vi "Test Line Result.vi"(5 "Etalon number":u32, 7 "Ignore Error":bool, 8 "error in (no error)":errorcluster, 9 "Teszt cluster":T1, 10 "Thread ID":u16, 11 "Queue in":refnum<queue>) -> (0 "error out":errorcluster, 1 "Abort":bool, 2 "Etalon Kiértékelés":bool, 3 "Kiértékelés":bool)   [LabVIEW 2014]
uses:
  Teszt/Teszt.ctl
  Teszt/Command.ctl
  support/Message Queue/Message Cluster.ctl
  Message.ctl
  support/Message Queue/Enqueue Message (Single).vi
  support/Message Queue/Message Queue.lvlib
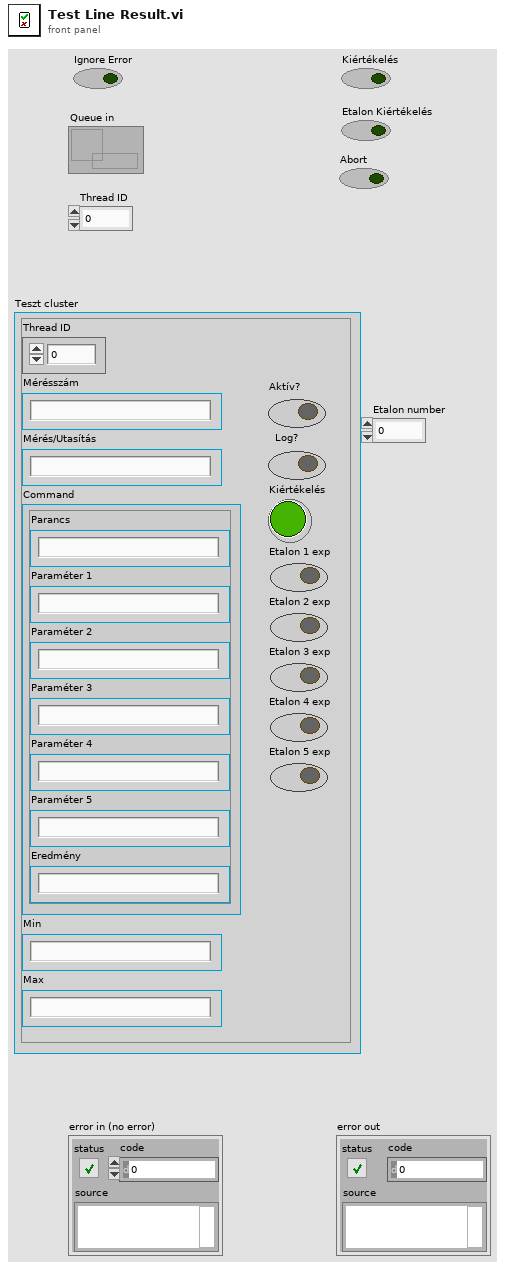
[diagram p1: front panel]
types:
  T1 = typedef "Teszt.ctl" = cluster{"Thread ID":dbl, "Mérésszám":string, "Mérés/Utasítás":string, "Command":T2, "Min":string, "Max":string, "Aktív?":bool, "Log?":bool, "Kiértékelés":bool, "Etalon 1 exp":bool, "Etalon 2 exp":bool, "Etalon 3 exp":bool, "Etalon 4 exp":bool, "Etalon 5 exp":bool}
  T2 = typedef "Command.ctl" = cluster{"Parancs":string, "Paraméter 1":string, "Paraméter 2":string, "Paraméter 3":string, "Paraméter 4":string, "Paraméter 5":string, "Eredmény":string}
  T3 = typedef "Message.ctl" = cluster{"Thread ID":u16, "Callback":string, "Data":variant, "Error":errorcluster}
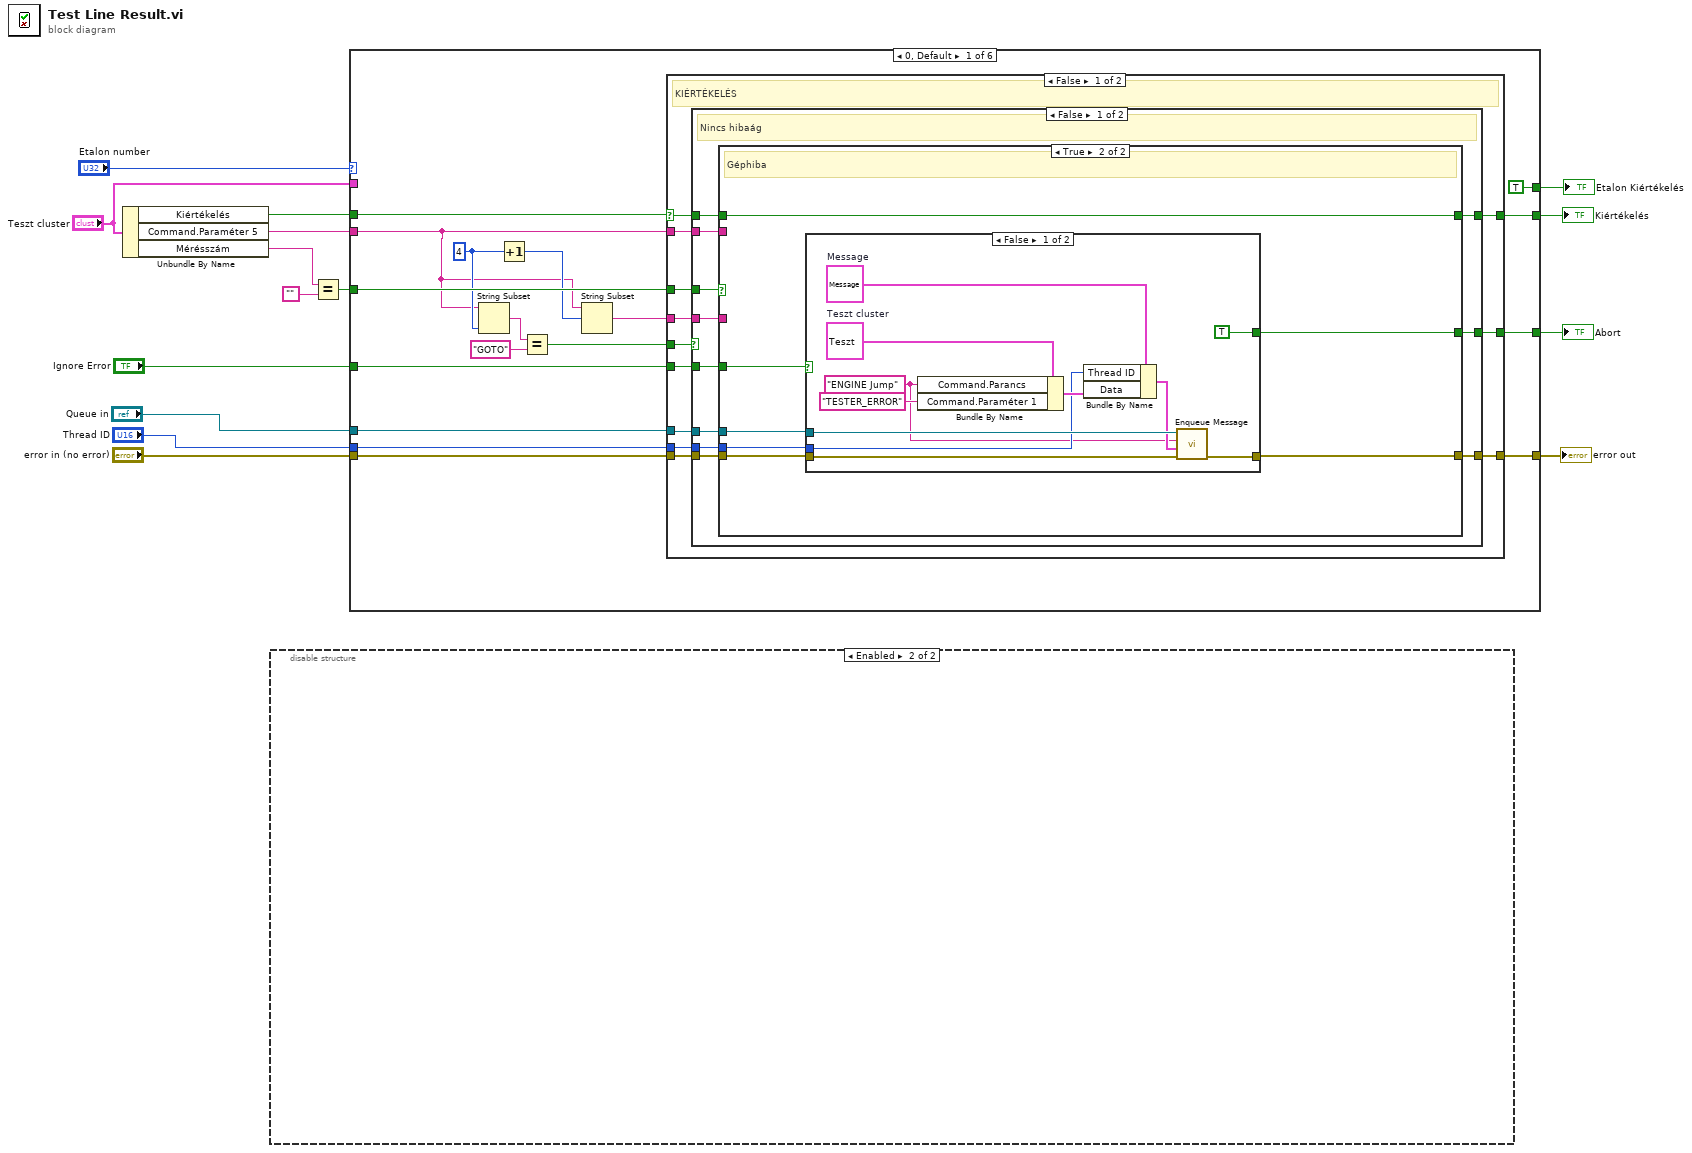
[diagram p0: block diagram]
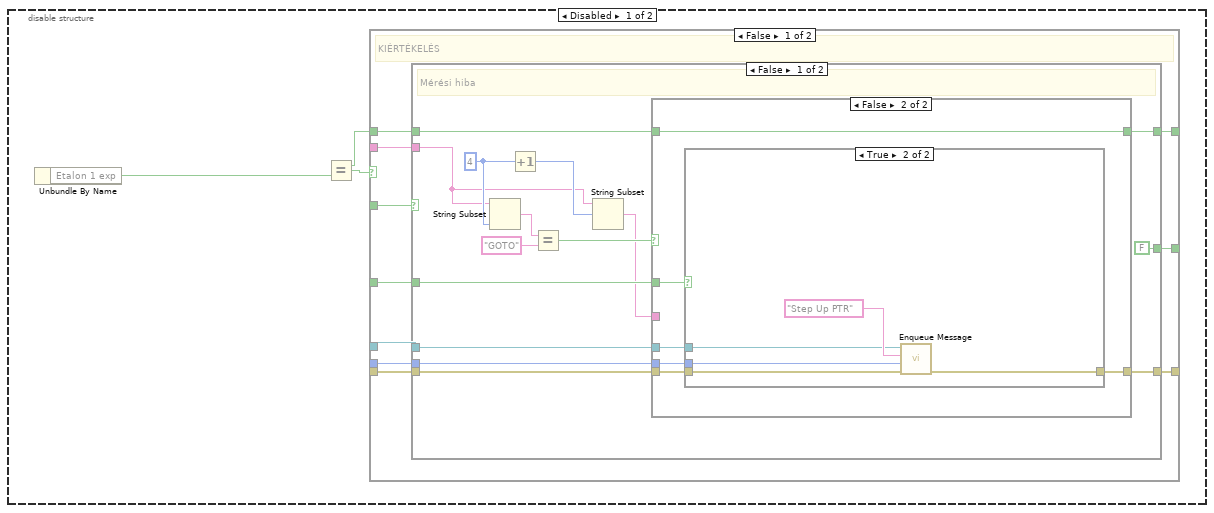
[diagram p2: hidden frame]
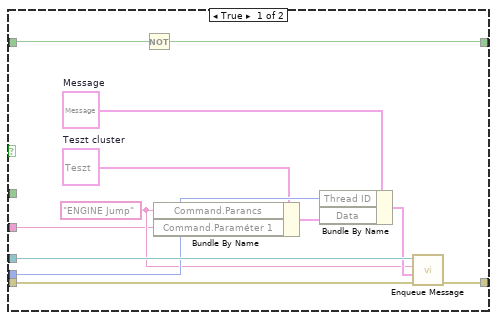
[diagram p3: hidden frame]
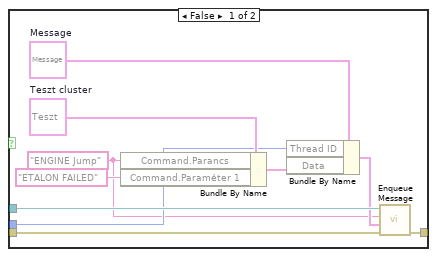
[diagram p4: hidden frame]
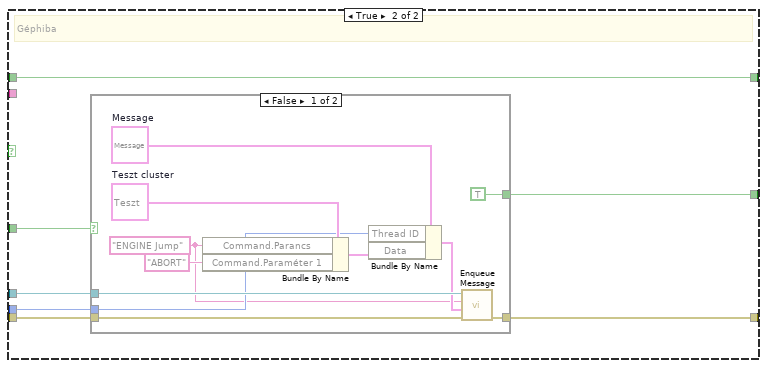
[diagram p5: hidden frame]
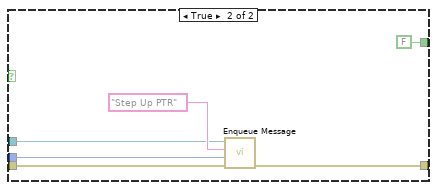
[diagram p6: hidden frame]
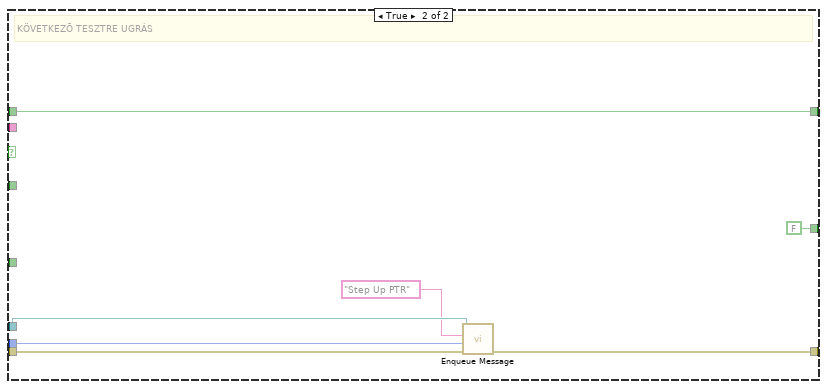
[diagram p7: hidden frame]
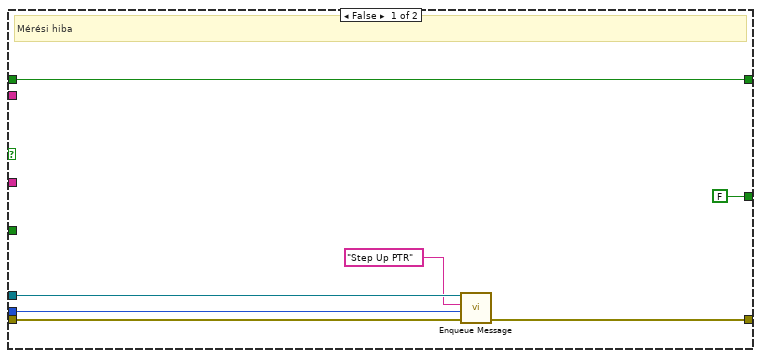
[diagram p8: hidden frame]
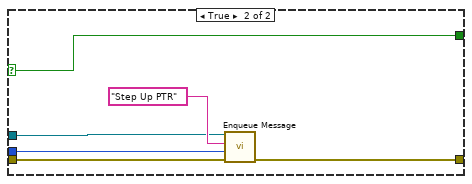
[diagram p9: hidden frame]
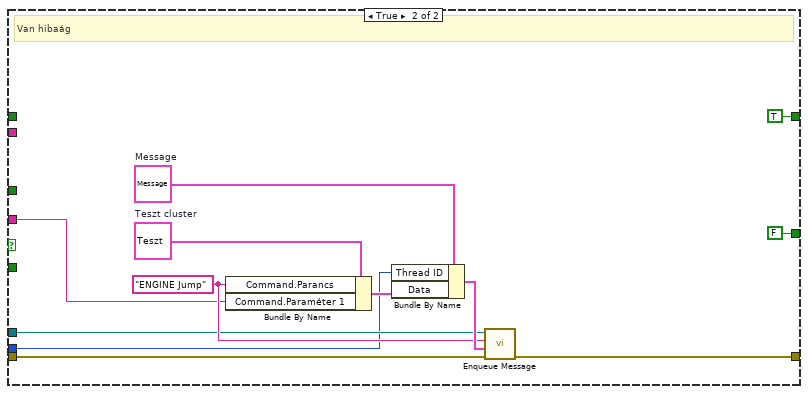
[diagram p10: hidden frame]
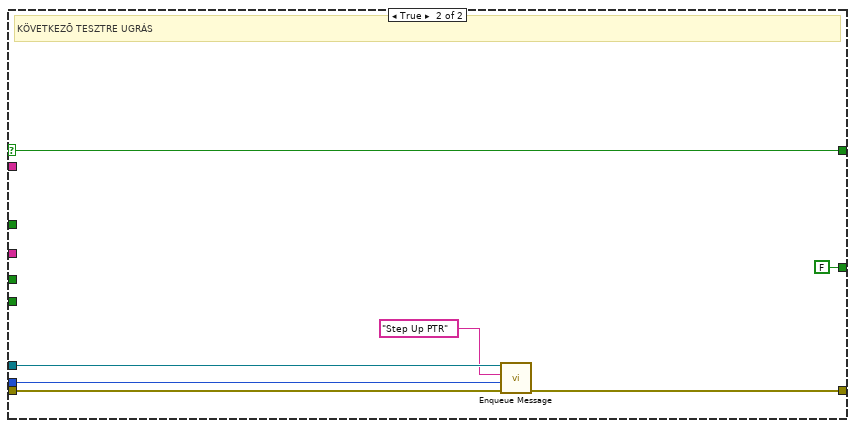
[diagram p11: hidden frame]
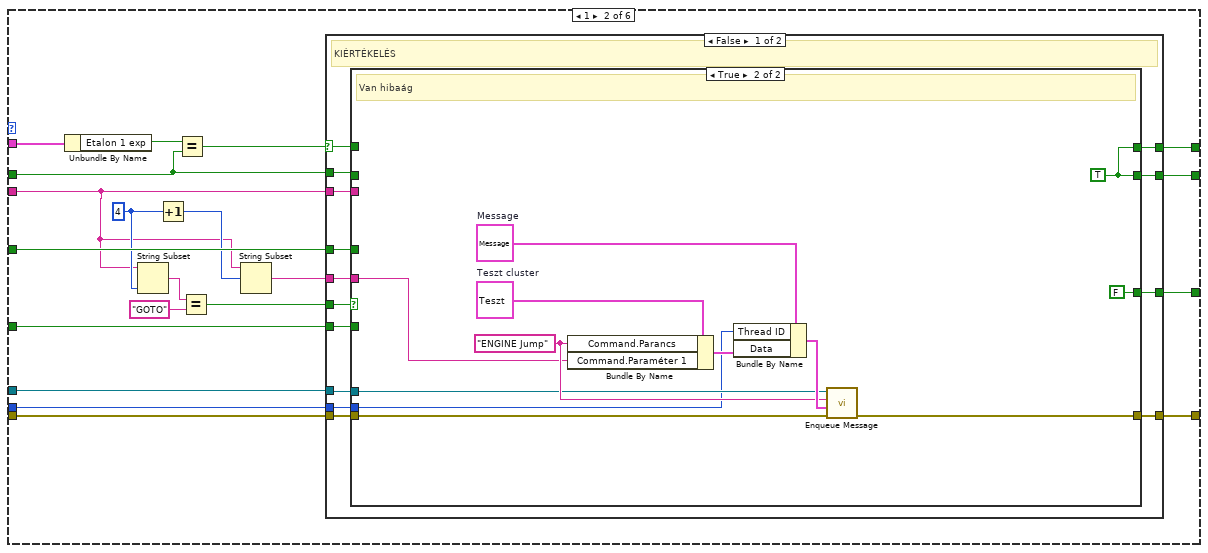
[diagram p12: hidden frame]
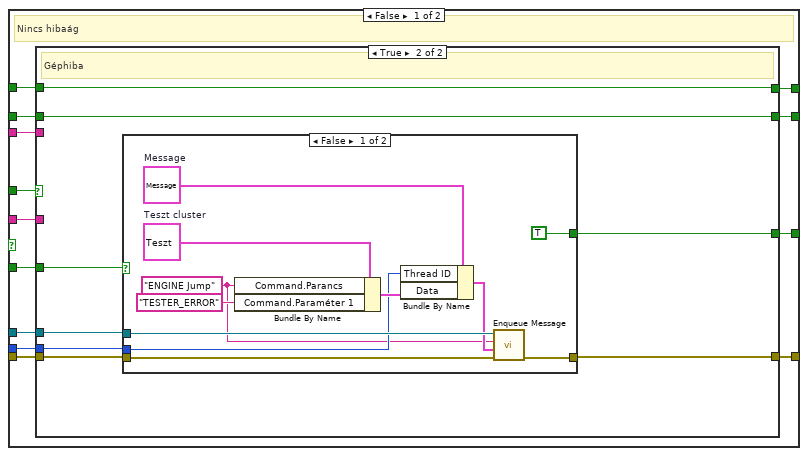
[diagram p13: hidden frame]
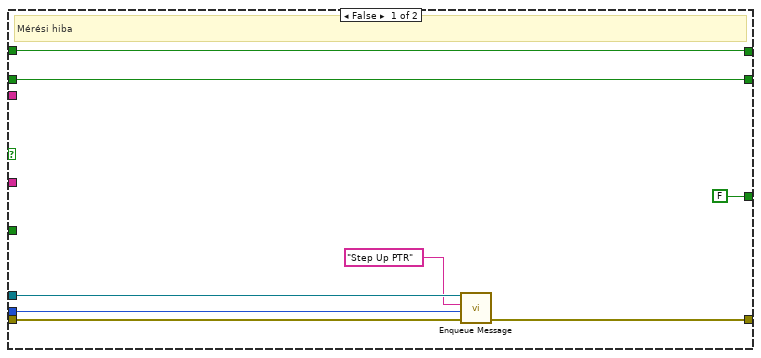
[diagram p14: hidden frame]
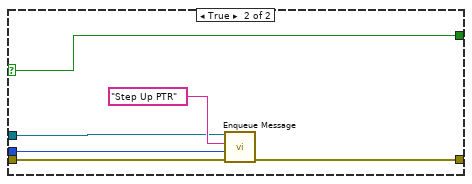
[diagram p15: hidden frame]
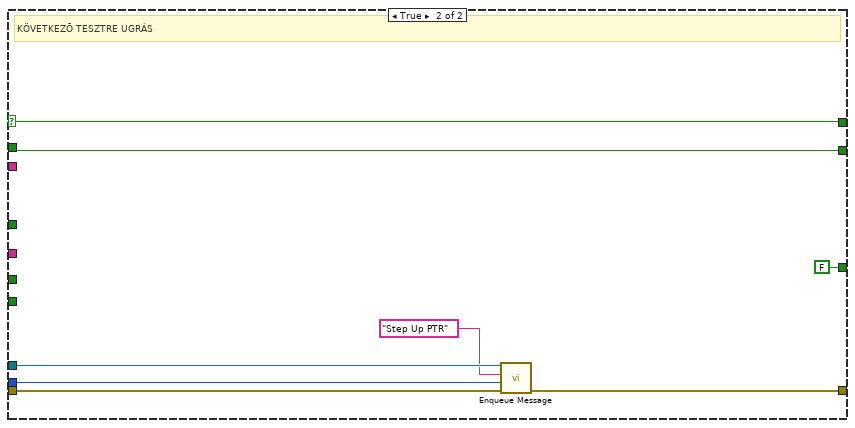
[diagram p16: hidden frame]
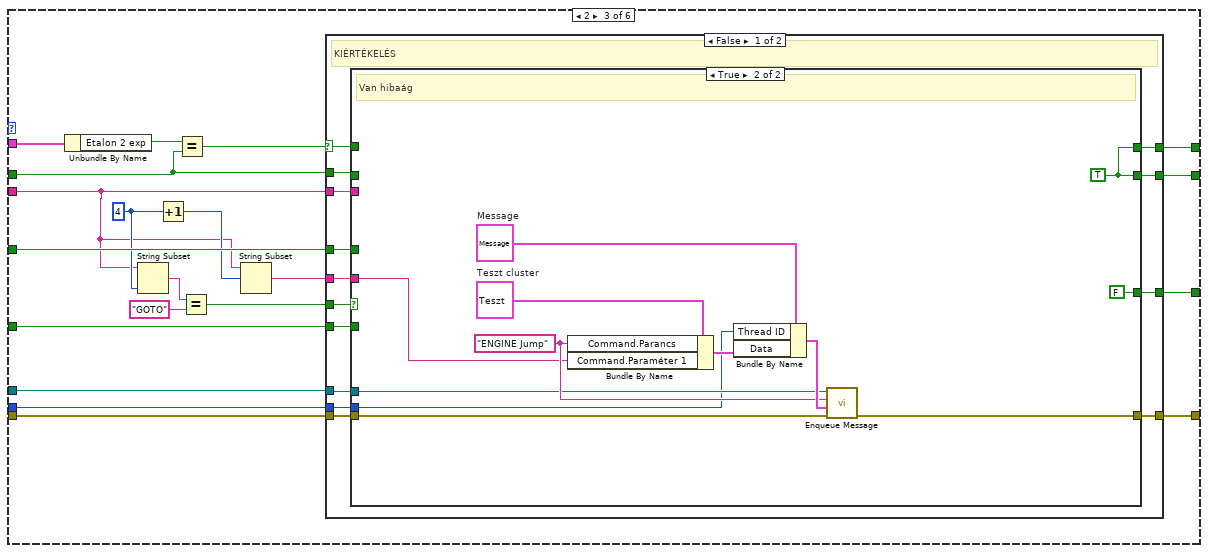
[diagram p17: hidden frame]
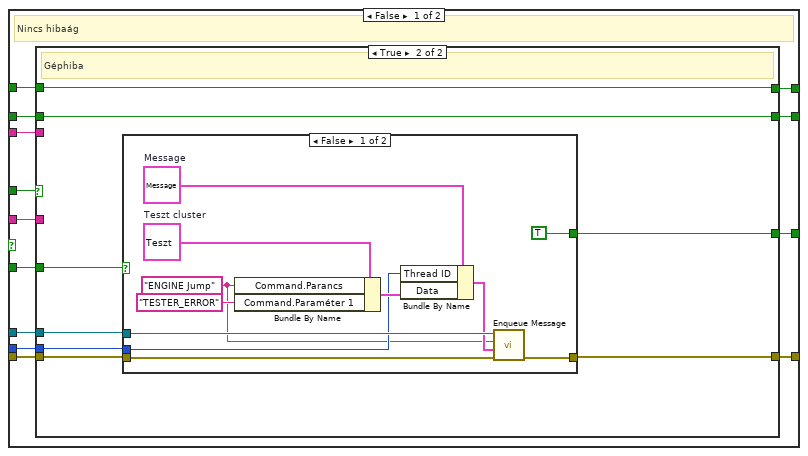
[diagram p18: hidden frame]
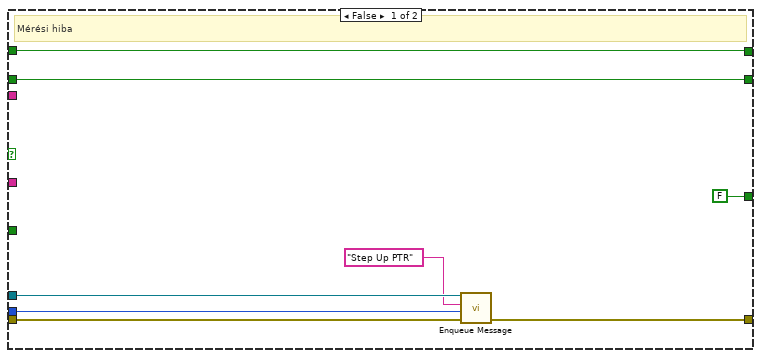
[diagram p19: hidden frame]
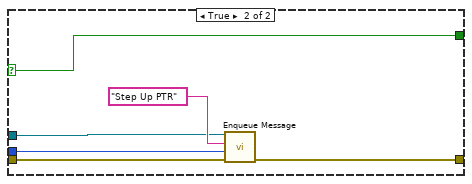
[diagram p20: hidden frame]
diagram:
  n1 = Unbundle By Name("Teszt cluster") -> ("Kiértékelés"=w11:bool, "Command.Paraméter 5"=w8:string, "Mérésszám"=w5:string)
  n2 = disable-structure shown="Enabled" {
    frame Disabled {
      n3 = Unbundle By Name() -> ("Etalon 1 exp"=w20:bool)  [unwired: 1 in]
      n4 = Equal?(y=w20) -> (x=w21:bool, x = y?=w23:bool)
      n5 = case shown="False" w23 {
        tunnel: [w34 w113] -> _
        tunnel: [w33 w112] -> w16
        tunnel: [w32 w111] -> w17
        tunnel: [w30 w109] -> w18
        tunnel: [w31 _] -> w22
        tunnel: [w28 w108] -> _
        tunnel: [w29 _] -> w19
        tunnel: w21 -> [w27 w108]
        tunnel: [w26 _] -> w24
        tunnel: [w25 FALSE] -> _
        frame False {
          # "KIÉRTÉKELÉS"
          n6 = case shown="False" w26 {
            tunnel: [w49 w85] -> w34
            tunnel: w33 -> [w48 w89]
            tunnel: w32 -> [w47 w87]
            tunnel: w31 -> [w46 w86]
            tunnel: w30 -> [w45 w88]
            tunnel: w29 -> [w40 _]
            tunnel: [w37 w84] -> w28
            tunnel: w27 -> [w36 w84]
            tunnel: [FALSE w83] -> w25
            frame False {
              w43 = 4 ("length (rest)")
              # "Mérési hiba"
              n7 = String Subset(string=w40, length (rest)=w43) -> (substring=w41:string)  [unwired: 1 in]
              n8 = Increment(x=w43) -> (x+1=w44:i32)
              n9 = Equal?(x=w41, y="GOTO") -> (x = y?=w39:bool)
              n10 = String Subset(string=w40, offset (0)=w44) -> (substring=w38:string)  [unwired: 1 in]
              n11 = case shown="False" w39 {
                tunnel: [w61 w67] -> w49
                tunnel: w48 -> [w60 w66]
                tunnel: w47 -> [w59 w65]
                tunnel: w46 -> [_ w64]
                tunnel: w45 -> [w58 w63]
                tunnel: w38 -> [w52 _]
                tunnel: w36 -> [w51 w62]
                tunnel: [w50 w62] -> w37
                frame True {
                  w53 = "ENGINE Jump" ("Command.Parancs")
                  w56 = T1 {"Thread ID"=0.0, "Mérésszám"="", "Mérés/Utasítás"="", "Command"={"Parancs"="", "Paraméter 1"="", "Paraméter 2"="", "Paraméter 3"="", "Paraméter 4"="", "Paraméter 5"="", "Eredmény"=""}, "Min"="", "Max"="", "Aktív?"=FALSE, "Log?"=FALSE, "Kiértékelés"=FALSE, "Etalon 1 exp"=FALSE, "Etalon 2 exp"=FALSE, "Etalon 3 exp"=FALSE, "Etalon 4 exp"=FALSE, "Etalon 5 exp"=FALSE}  # Teszt cluster
                  w55 = T3 {"Thread ID"=0, "Callback"="", "Data"=variant, "Error"={"status"=FALSE, "code"=0, "source"=""}}  # Message
                  n12 = Not(x=w51) -> (.not. x?=w50:bool)
                  n13 = Bundle By Name(cluster=w56, "Command.Parancs"=w53, "Command.Paraméter 1"=w52) -> (w57:T1)
                  n14 = Bundle By Name(cluster=w55, "Thread ID"=w58, "Data"=w57) -> (w54:T3)
                  n15 = call-poly "Enqueue Message.vi"("error in (no error)"=w60, "Message Data"=w54, "Message"=w53, "Message Queue"=w59) -> ("error out"=w61:errorcluster)  [unwired: 6 in, 1 out]
                }
                frame False {
                  n16 = case shown="True" w64 {
                    tunnel: [w77 w78] -> w67
                    tunnel: w66 -> [w76 w80]
                    tunnel: w65 -> [w75 w81]
                    tunnel: w63 -> [w69 w79]
                    frame False {
                      w68 = "ENGINE Jump" ("Command.Parancs")
                      w72 = T1 {"Thread ID"=0.0, "Mérésszám"="", "Mérés/Utasítás"="", "Command"={"Parancs"="", "Paraméter 1"="", "Paraméter 2"="", "Paraméter 3"="", "Paraméter 4"="", "Paraméter 5"="", "Eredmény"=""}, "Min"="", "Max"="", "Aktív?"=FALSE, "Log?"=FALSE, "Kiértékelés"=FALSE, "Etalon 1 exp"=FALSE, "Etalon 2 exp"=FALSE, "Etalon 3 exp"=FALSE, "Etalon 4 exp"=FALSE, "Etalon 5 exp"=FALSE}  # Teszt cluster
                      w71 = T3 {"Thread ID"=0, "Callback"="", "Data"=variant, "Error"={"status"=FALSE, "code"=0, "source"=""}}  # Message
                      n17 = Bundle By Name(cluster=w72, "Command.Parancs"=w68, "Command.Paraméter 1"="ETALON FAILED") -> (w74:T1)
                      n18 = Bundle By Name(cluster=w71, "Thread ID"=w69, "Data"=w74) -> (w70:T3)
                      n19 = call-poly "Enqueue Message.vi"("error in (no error)"=w76, "Message Data"=w70, "Message"=w68, "Message Queue"=w75) -> ("error out"=w77:errorcluster)  [unwired: 6 in, 1 out]
                    }
                    frame True {
                      n20 = call-poly "Enqueue Message.vi"("error in (no error)"=w80, "Message Data"=w79, "Message"="Step Up PTR", "Message Queue"=w81) -> ("error out"=w78:errorcluster)  [unwired: 6 in, 1 out]
                    }
                  }
                }
              }
            }
            frame True {
              # "Géphiba"
              n21 = case shown="False" w86 {
                tunnel: [w100 w102] -> w85
                tunnel: w89 -> [w99 w104]
                tunnel: w87 -> [w98 w105]
                tunnel: w88 -> [w92 w103]
                tunnel: [TRUE FALSE] -> w83
                frame False {
                  w91 = "ENGINE Jump" ("Command.Parancs")
                  w95 = T1 {"Thread ID"=0.0, "Mérésszám"="", "Mérés/Utasítás"="", "Command"={"Parancs"="", "Paraméter 1"="", "Paraméter 2"="", "Paraméter 3"="", "Paraméter 4"="", "Paraméter 5"="", "Eredmény"=""}, "Min"="", "Max"="", "Aktív?"=FALSE, "Log?"=FALSE, "Kiértékelés"=FALSE, "Etalon 1 exp"=FALSE, "Etalon 2 exp"=FALSE, "Etalon 3 exp"=FALSE, "Etalon 4 exp"=FALSE, "Etalon 5 exp"=FALSE}  # Teszt cluster
                  w94 = T3 {"Thread ID"=0, "Callback"="", "Data"=variant, "Error"={"status"=FALSE, "code"=0, "source"=""}}  # Message
                  n22 = Bundle By Name(cluster=w95, "Command.Parancs"=w91, "Command.Paraméter 1"="ABORT") -> (w97:T1)
                  n23 = Bundle By Name(cluster=w94, "Thread ID"=w92, "Data"=w97) -> (w93:T3)
                  n24 = call-poly "Enqueue Message.vi"("error in (no error)"=w99, "Message Data"=w93, "Message"=w91, "Message Queue"=w98) -> ("error out"=w100:errorcluster)  [unwired: 6 in, 1 out]
                }
                frame True {
                  n25 = call-poly "Enqueue Message.vi"("error in (no error)"=w104, "Message Data"=w103, "Message"="Step Up PTR", "Message Queue"=w105) -> ("error out"=w102:errorcluster)  [unwired: 6 in, 1 out]
                }
              }
            }
          }
        }
        frame True {
          # "KÖVETKEZÕ TESZTRE UGRÁS"
          n26 = call-poly "Enqueue Message.vi"("error in (no error)"=w112, "Message Data"=w109, "Message"="Step Up PTR", "Message Queue"=w111) -> ("error out"=w113:errorcluster)  [unwired: 6 in, 1 out]
        }
      }
    }
    frame Enabled {
    }
  }
  n27 = Equal?(x=w5, y="") -> (x = y?=w3:bool)
  n28 = case shown="0, Default" "Etalon number" {
    tunnel: [w130 w223 w323 w423 w523 w623] -> w15
    tunnel: "error in (no error)" -> [w129 w222 w322 w422 w522 w622]
    tunnel: "Ignore Error" -> [w128 w221 w321 w421 w521 w621]
    tunnel: "Thread ID" -> [w127 w220 w320 w420 w520 w620]
    tunnel: w11 -> [w126 w205 w305 w405 w505 w605]
    tunnel: "Queue in" -> [w125 w219 w319 w419 w519 w619]
    tunnel: [w124 w218 w318 w418 w518 w618] -> w9
    tunnel: w8 -> [w117 w211 w311 w411 w511 w611]
    tunnel: "Teszt cluster" -> [_ w208 w308 w408 w508 w608]
    tunnel: w3 -> [w123 w217 w317 w417 w517 w617]
    tunnel: [w122 w216 w316 w416 w516 w616] -> w2
    tunnel: [TRUE w204 w304 w404 w504 w604] -> w1
    frame 0, Default {
      w119 = 4 ("length (rest)")
      n29 = String Subset(string=w117, length (rest)=w119) -> (substring=w121:string)  [unwired: 1 in]
      n30 = Increment(x=w119) -> (x+1=w118:i32)
      n31 = Equal?(x=w121, y="GOTO") -> (x = y?=w116:bool)
      n32 = String Subset(string=w117, offset (0)=w118) -> (substring=w115:string)  [unwired: 1 in]
      n33 = case shown="False" w126 {
        selector: w126 -> [w136 w198]
        tunnel: [w142 w203] -> w124
        tunnel: w129 -> [w141 w202]
        tunnel: w125 -> [w140 w201]
        tunnel: w127 -> [w138 w199]
        tunnel: w128 -> [w139 _]
        tunnel: [w135 w198] -> w130
        tunnel: w117 -> [w137 _]
        tunnel: w123 -> [w134 _]
        tunnel: [w133 FALSE] -> w122
        tunnel: w116 -> [w131 _]
        tunnel: w115 -> [w132 _]
        frame False {
          # "KIÉRTÉKELÉS"
          n34 = case shown="False" w131 {
            tunnel: [w153 w188] -> w142
            tunnel: w141 -> [w152 w189]
            tunnel: w140 -> [w151 w191]
            tunnel: w139 -> [w150 _]
            tunnel: w138 -> [w149 w190]
            tunnel: w137 -> [w148 _]
            tunnel: w136 -> [w147 _]
            tunnel: [w146 TRUE] -> w135
            tunnel: w134 -> [w145 _]
            tunnel: [w144 FALSE] -> w133
            tunnel: w132 -> [w143 w187]
            frame False {
              # "Nincs hibaág"
              n35 = case shown="True" w145 {
                tunnel: [w160 w163] -> w153
                tunnel: w152 -> [w159 w164]
                tunnel: w151 -> [w158 w166]
                tunnel: w150 -> [_ w161]
                tunnel: w149 -> [w157 w165]
                tunnel: w148 -> [_ _]
                tunnel: w147 -> [w156 w167]
                tunnel: [w156 w167] -> w146
                tunnel: [FALSE w162] -> w144
                tunnel: w143 -> [_ _]
                frame False {
                  # "Mérési hiba"
                  n36 = call-poly "Enqueue Message.vi"("error in (no error)"=w159, "Message Data"=w157, "Message"="Step Up PTR", "Message Queue"=w158) -> ("error out"=w160:errorcluster)  [unwired: 6 in, 1 out]
                }
                frame True {
                  # "Géphiba"
                  n37 = case shown="False" w161 {
                    selector: w161 -> [_ w179]
                    tunnel: [w178 w180] -> w163
                    tunnel: w164 -> [w177 w182]
                    tunnel: w166 -> [w176 w183]
                    tunnel: w165 -> [w170 w181]
                    tunnel: [TRUE w179] -> w162
                    frame False {
                      w169 = "ENGINE Jump" ("Command.Parancs")
                      w173 = T1 {"Thread ID"=0.0, "Mérésszám"="", "Mérés/Utasítás"="", "Command"={"Parancs"="", "Paraméter 1"="", "Paraméter 2"="", "Paraméter 3"="", "Paraméter 4"="", "Paraméter 5"="", "Eredmény"=""}, "Min"="", "Max"="", "Aktív?"=FALSE, "Log?"=FALSE, "Kiértékelés"=FALSE, "Etalon 1 exp"=FALSE, "Etalon 2 exp"=FALSE, "Etalon 3 exp"=FALSE, "Etalon 4 exp"=FALSE, "Etalon 5 exp"=FALSE}  # Teszt cluster
                      w172 = T3 {"Thread ID"=0, "Callback"="", "Data"=variant, "Error"={"status"=FALSE, "code"=0, "source"=""}}  # Message
                      n38 = Bundle By Name(cluster=w173, "Command.Parancs"=w169, "Command.Paraméter 1"="TESTER_ERROR") -> (w175:T1)
                      n39 = Bundle By Name(cluster=w172, "Thread ID"=w170, "Data"=w175) -> (w171:T3)
                      n40 = call-poly "Enqueue Message.vi"("error in (no error)"=w177, "Message Data"=w171, "Message"=w169, "Message Queue"=w176) -> ("error out"=w178:errorcluster)  [unwired: 6 in, 1 out]
                    }
                    frame True {
                      n41 = call-poly "Enqueue Message.vi"("error in (no error)"=w182, "Message Data"=w181, "Message"="Step Up PTR", "Message Queue"=w183) -> ("error out"=w180:errorcluster)  [unwired: 6 in, 1 out]
                    }
                  }
                }
              }
            }
            frame True {
              w192 = "ENGINE Jump" ("Command.Parancs")
              w195 = T1 {"Thread ID"=0.0, "Mérésszám"="", "Mérés/Utasítás"="", "Command"={"Parancs"="", "Paraméter 1"="", "Paraméter 2"="", "Paraméter 3"="", "Paraméter 4"="", "Paraméter 5"="", "Eredmény"=""}, "Min"="", "Max"="", "Aktív?"=FALSE, "Log?"=FALSE, "Kiértékelés"=FALSE, "Etalon 1 exp"=FALSE, "Etalon 2 exp"=FALSE, "Etalon 3 exp"=FALSE, "Etalon 4 exp"=FALSE, "Etalon 5 exp"=FALSE}  # Teszt cluster
              w194 = T3 {"Thread ID"=0, "Callback"="", "Data"=variant, "Error"={"status"=FALSE, "code"=0, "source"=""}}  # Message
              # "Van hibaág"
              n42 = Bundle By Name(cluster=w195, "Command.Parancs"=w192, "Command.Paraméter 1"=w187) -> (w196:T1)
              n43 = Bundle By Name(cluster=w194, "Thread ID"=w190, "Data"=w196) -> (w193:T3)
              n44 = call-poly "Enqueue Message.vi"("error in (no error)"=w189, "Message Data"=w193, "Message"=w192, "Message Queue"=w191) -> ("error out"=w188:errorcluster)  [unwired: 6 in, 1 out]
            }
          }
        }
        frame True {
          # "KÖVETKEZÕ TESZTRE UGRÁS"
          n45 = call-poly "Enqueue Message.vi"("error in (no error)"=w202, "Message Data"=w199, "Message"="Step Up PTR", "Message Queue"=w201) -> ("error out"=w203:errorcluster)  [unwired: 6 in, 1 out]
        }
      }
    }
    frame 1 {
      w213 = 4 ("length (rest)")
      n46 = Unbundle By Name(w208) -> ("Etalon 1 exp"=w207:bool)
      n47 = String Subset(string=w211, length (rest)=w213) -> (substring=w215:string)  [unwired: 1 in]
      n48 = Increment(x=w213) -> (x+1=w212:i32)
      n49 = Equal?(x=w207, y=w205) -> (x = y?=w206:bool)
      n50 = Equal?(x=w215, y="GOTO") -> (x = y?=w210:bool)
      n51 = String Subset(string=w211, offset (0)=w212) -> (substring=w209:string)  [unwired: 1 in]
      n52 = case shown="False" w206 {
        selector: w206 -> [w225 w296]
        tunnel: [w237 w303] -> w218
        tunnel: w222 -> [w236 w302]
        tunnel: w219 -> [w235 w301]
        tunnel: w220 -> [w233 w299]
        tunnel: w221 -> [w234 _]
        tunnel: [w231 w297] -> w223
        tunnel: w211 -> [w232 _]
        tunnel: w217 -> [w230 _]
        tunnel: [w229 FALSE] -> w216
        tunnel: w210 -> [w227 _]
        tunnel: w209 -> [w228 _]
        tunnel: w205 -> [w226 w297]
        tunnel: [w224 w296] -> w204
        frame False {
          # "KIÉRTÉKELÉS"
          n53 = case shown="True" w227 {
            tunnel: [w250 w287] -> w237
            tunnel: w236 -> [w249 w288]
            tunnel: w235 -> [w248 w290]
            tunnel: w234 -> [w247 _]
            tunnel: w233 -> [w246 w289]
            tunnel: w232 -> [w245 _]
            tunnel: w226 -> [w244 _]
            tunnel: [w243 w284] -> w231
            tunnel: w230 -> [w242 _]
            tunnel: [w241 FALSE] -> w229
            tunnel: w228 -> [w240 w286]
            tunnel: w225 -> [w239 _]
            tunnel: [w238 w284] -> w224
            frame False {
              # "Nincs hibaág"
              n54 = case shown="True" w242 {
                tunnel: [w258 w262] -> w250
                tunnel: w249 -> [w257 w263]
                tunnel: w248 -> [w256 w265]
                tunnel: w247 -> [_ w260]
                tunnel: w246 -> [w255 w264]
                tunnel: w245 -> [_ _]
                tunnel: w244 -> [w254 w266]
                tunnel: [w254 w266] -> w243
                tunnel: [FALSE w261] -> w241
                tunnel: w240 -> [_ _]
                tunnel: w239 -> [w251 w259]
                tunnel: [w251 w259] -> w238
                frame False {
                  # "Mérési hiba"
                  n55 = call-poly "Enqueue Message.vi"("error in (no error)"=w257, "Message Data"=w255, "Message"="Step Up PTR", "Message Queue"=w256) -> ("error out"=w258:errorcluster)  [unwired: 6 in, 1 out]
                }
                frame True {
                  # "Géphiba"
                  n56 = case shown="False" w260 {
                    selector: w260 -> [_ w278]
                    tunnel: [w277 w279] -> w262
                    tunnel: w263 -> [w276 w281]
                    tunnel: w265 -> [w275 w282]
                    tunnel: w264 -> [w269 w280]
                    tunnel: [TRUE w278] -> w261
                    frame False {
                      w268 = "ENGINE Jump" ("Command.Parancs")
                      w272 = T1 {"Thread ID"=0.0, "Mérésszám"="", "Mérés/Utasítás"="", "Command"={"Parancs"="", "Paraméter 1"="", "Paraméter 2"="", "Paraméter 3"="", "Paraméter 4"="", "Paraméter 5"="", "Eredmény"=""}, "Min"="", "Max"="", "Aktív?"=FALSE, "Log?"=FALSE, "Kiértékelés"=FALSE, "Etalon 1 exp"=FALSE, "Etalon 2 exp"=FALSE, "Etalon 3 exp"=FALSE, "Etalon 4 exp"=FALSE, "Etalon 5 exp"=FALSE}  # Teszt cluster
                      w271 = T3 {"Thread ID"=0, "Callback"="", "Data"=variant, "Error"={"status"=FALSE, "code"=0, "source"=""}}  # Message
                      n57 = Bundle By Name(cluster=w272, "Command.Parancs"=w268, "Command.Paraméter 1"="TESTER_ERROR") -> (w274:T1)
                      n58 = Bundle By Name(cluster=w271, "Thread ID"=w269, "Data"=w274) -> (w270:T3)
                      n59 = call-poly "Enqueue Message.vi"("error in (no error)"=w276, "Message Data"=w270, "Message"=w268, "Message Queue"=w275) -> ("error out"=w277:errorcluster)  [unwired: 6 in, 1 out]
                    }
                    frame True {
                      n60 = call-poly "Enqueue Message.vi"("error in (no error)"=w281, "Message Data"=w280, "Message"="Step Up PTR", "Message Queue"=w282) -> ("error out"=w279:errorcluster)  [unwired: 6 in, 1 out]
                    }
                  }
                }
              }
            }
            frame True {
              w284 = TRUE
              w291 = "ENGINE Jump" ("Command.Parancs")
              w294 = T1 {"Thread ID"=0.0, "Mérésszám"="", "Mérés/Utasítás"="", "Command"={"Parancs"="", "Paraméter 1"="", "Paraméter 2"="", "Paraméter 3"="", "Paraméter 4"="", "Paraméter 5"="", "Eredmény"=""}, "Min"="", "Max"="", "Aktív?"=FALSE, "Log?"=FALSE, "Kiértékelés"=FALSE, "Etalon 1 exp"=FALSE, "Etalon 2 exp"=FALSE, "Etalon 3 exp"=FALSE, "Etalon 4 exp"=FALSE, "Etalon 5 exp"=FALSE}  # Teszt cluster
              w293 = T3 {"Thread ID"=0, "Callback"="", "Data"=variant, "Error"={"status"=FALSE, "code"=0, "source"=""}}  # Message
              # "Van hibaág"
              n61 = Bundle By Name(cluster=w294, "Command.Parancs"=w291, "Command.Paraméter 1"=w286) -> (w295:T1)
              n62 = Bundle By Name(cluster=w293, "Thread ID"=w289, "Data"=w295) -> (w292:T3)
              n63 = call-poly "Enqueue Message.vi"("error in (no error)"=w288, "Message Data"=w292, "Message"=w291, "Message Queue"=w290) -> ("error out"=w287:errorcluster)  [unwired: 6 in, 1 out]
            }
          }
        }
        frame True {
          # "KÖVETKEZÕ TESZTRE UGRÁS"
          n64 = call-poly "Enqueue Message.vi"("error in (no error)"=w302, "Message Data"=w299, "Message"="Step Up PTR", "Message Queue"=w301) -> ("error out"=w303:errorcluster)  [unwired: 6 in, 1 out]
        }
      }
    }
    frame 2 {
      w313 = 4 ("length (rest)")
      n65 = Unbundle By Name(w308) -> ("Etalon 2 exp"=w307:bool)
      n66 = String Subset(string=w311, length (rest)=w313) -> (substring=w315:string)  [unwired: 1 in]
      n67 = Increment(x=w313) -> (x+1=w312:i32)
      n68 = Equal?(x=w307, y=w305) -> (x = y?=w306:bool)
      n69 = Equal?(x=w315, y="GOTO") -> (x = y?=w310:bool)
      n70 = String Subset(string=w311, offset (0)=w312) -> (substring=w309:string)  [unwired: 1 in]
      n71 = case shown="False" w306 {
        selector: w306 -> [w325 w396]
        tunnel: [w337 w403] -> w318
        tunnel: w322 -> [w336 w402]
        tunnel: w319 -> [w335 w401]
        tunnel: w320 -> [w333 w399]
        tunnel: w321 -> [w334 _]
        tunnel: [w331 w397] -> w323
        tunnel: w311 -> [w332 _]
        tunnel: w317 -> [w330 _]
        tunnel: [w329 FALSE] -> w316
        tunnel: w310 -> [w327 _]
        tunnel: w309 -> [w328 _]
        tunnel: w305 -> [w326 w397]
        tunnel: [w324 w396] -> w304
        frame False {
          # "KIÉRTÉKELÉS"
          n72 = case shown="True" w327 {
            tunnel: [w350 w387] -> w337
            tunnel: w336 -> [w349 w388]
            tunnel: w335 -> [w348 w390]
            tunnel: w334 -> [w347 _]
            tunnel: w333 -> [w346 w389]
            tunnel: w332 -> [w345 _]
            tunnel: w326 -> [w344 _]
            tunnel: [w343 w384] -> w331
            tunnel: w330 -> [w342 _]
            tunnel: [w341 FALSE] -> w329
            tunnel: w328 -> [w340 w386]
            tunnel: w325 -> [w339 _]
            tunnel: [w338 w384] -> w324
            frame False {
              # "Nincs hibaág"
              n73 = case shown="True" w342 {
                tunnel: [w358 w362] -> w350
                tunnel: w349 -> [w357 w363]
                tunnel: w348 -> [w356 w365]
                tunnel: w347 -> [_ w360]
                tunnel: w346 -> [w355 w364]
                tunnel: w345 -> [_ _]
                tunnel: w344 -> [w354 w366]
                tunnel: [w354 w366] -> w343
                tunnel: [FALSE w361] -> w341
                tunnel: w340 -> [_ _]
                tunnel: w339 -> [w351 w359]
                tunnel: [w351 w359] -> w338
                frame False {
                  # "Mérési hiba"
                  n74 = call-poly "Enqueue Message.vi"("error in (no error)"=w357, "Message Data"=w355, "Message"="Step Up PTR", "Message Queue"=w356) -> ("error out"=w358:errorcluster)  [unwired: 6 in, 1 out]
                }
                frame True {
                  # "Géphiba"
                  n75 = case shown="False" w360 {
                    selector: w360 -> [_ w378]
                    tunnel: [w377 w379] -> w362
                    tunnel: w363 -> [w376 w381]
                    tunnel: w365 -> [w375 w382]
                    tunnel: w364 -> [w369 w380]
                    tunnel: [TRUE w378] -> w361
                    frame False {
                      w368 = "ENGINE Jump" ("Command.Parancs")
                      w372 = T1 {"Thread ID"=0.0, "Mérésszám"="", "Mérés/Utasítás"="", "Command"={"Parancs"="", "Paraméter 1"="", "Paraméter 2"="", "Paraméter 3"="", "Paraméter 4"="", "Paraméter 5"="", "Eredmény"=""}, "Min"="", "Max"="", "Aktív?"=FALSE, "Log?"=FALSE, "Kiértékelés"=FALSE, "Etalon 1 exp"=FALSE, "Etalon 2 exp"=FALSE, "Etalon 3 exp"=FALSE, "Etalon 4 exp"=FALSE, "Etalon 5 exp"=FALSE}  # Teszt cluster
                      w371 = T3 {"Thread ID"=0, "Callback"="", "Data"=variant, "Error"={"status"=FALSE, "code"=0, "source"=""}}  # Message
                      n76 = Bundle By Name(cluster=w372, "Command.Parancs"=w368, "Command.Paraméter 1"="TESTER_ERROR") -> (w374:T1)
                      n77 = Bundle By Name(cluster=w371, "Thread ID"=w369, "Data"=w374) -> (w370:T3)
                      n78 = call-poly "Enqueue Message.vi"("error in (no error)"=w376, "Message Data"=w370, "Message"=w368, "Message Queue"=w375) -> ("error out"=w377:errorcluster)  [unwired: 6 in, 1 out]
                    }
                    frame True {
                      n79 = call-poly "Enqueue Message.vi"("error in (no error)"=w381, "Message Data"=w380, "Message"="Step Up PTR", "Message Queue"=w382) -> ("error out"=w379:errorcluster)  [unwired: 6 in, 1 out]
                    }
                  }
                }
              }
            }
            frame True {
              w384 = TRUE
              w391 = "ENGINE Jump" ("Command.Parancs")
              w394 = T1 {"Thread ID"=0.0, "Mérésszám"="", "Mérés/Utasítás"="", "Command"={"Parancs"="", "Paraméter 1"="", "Paraméter 2"="", "Paraméter 3"="", "Paraméter 4"="", "Paraméter 5"="", "Eredmény"=""}, "Min"="", "Max"="", "Aktív?"=FALSE, "Log?"=FALSE, "Kiértékelés"=FALSE, "Etalon 1 exp"=FALSE, "Etalon 2 exp"=FALSE, "Etalon 3 exp"=FALSE, "Etalon 4 exp"=FALSE, "Etalon 5 exp"=FALSE}  # Teszt cluster
              w393 = T3 {"Thread ID"=0, "Callback"="", "Data"=variant, "Error"={"status"=FALSE, "code"=0, "source"=""}}  # Message
              # "Van hibaág"
              n80 = Bundle By Name(cluster=w394, "Command.Parancs"=w391, "Command.Paraméter 1"=w386) -> (w395:T1)
              n81 = Bundle By Name(cluster=w393, "Thread ID"=w389, "Data"=w395) -> (w392:T3)
              n82 = call-poly "Enqueue Message.vi"("error in (no error)"=w388, "Message Data"=w392, "Message"=w391, "Message Queue"=w390) -> ("error out"=w387:errorcluster)  [unwired: 6 in, 1 out]
            }
          }
        }
        frame True {
          # "KÖVETKEZÕ TESZTRE UGRÁS"
          n83 = call-poly "Enqueue Message.vi"("error in (no error)"=w402, "Message Data"=w399, "Message"="Step Up PTR", "Message Queue"=w401) -> ("error out"=w403:errorcluster)  [unwired: 6 in, 1 out]
        }
      }
    }
    frame 3 {
      w413 = 4 ("length (rest)")
      n84 = Unbundle By Name(w408) -> ("Etalon 3 exp"=w407:bool)
      n85 = String Subset(string=w411, length (rest)=w413) -> (substring=w415:string)  [unwired: 1 in]
      n86 = Increment(x=w413) -> (x+1=w412:i32)
      n87 = Equal?(x=w407, y=w405) -> (x = y?=w406:bool)
      n88 = Equal?(x=w415, y="GOTO") -> (x = y?=w410:bool)
      n89 = String Subset(string=w411, offset (0)=w412) -> (substring=w409:string)  [unwired: 1 in]
      n90 = case shown="False" w406 {
        selector: w406 -> [w425 w496]
        tunnel: [w437 w503] -> w418
        tunnel: w422 -> [w436 w502]
        tunnel: w419 -> [w435 w501]
        tunnel: w420 -> [w433 w499]
        tunnel: w421 -> [w434 _]
        tunnel: [w431 w497] -> w423
        tunnel: w411 -> [w432 _]
        tunnel: w417 -> [w430 _]
        tunnel: [w429 FALSE] -> w416
        tunnel: w410 -> [w427 _]
        tunnel: w409 -> [w428 _]
        tunnel: w405 -> [w426 w497]
        tunnel: [w424 w496] -> w404
        frame False {
          # "KIÉRTÉKELÉS"
          n91 = case shown="True" w427 {
            tunnel: [w450 w487] -> w437
            tunnel: w436 -> [w449 w488]
            tunnel: w435 -> [w448 w490]
            tunnel: w434 -> [w447 _]
            tunnel: w433 -> [w446 w489]
            tunnel: w432 -> [w445 _]
            tunnel: w426 -> [w444 _]
            tunnel: [w443 w484] -> w431
            tunnel: w430 -> [w442 _]
            tunnel: [w441 FALSE] -> w429
            tunnel: w428 -> [w440 w486]
            tunnel: w425 -> [w439 _]
            tunnel: [w438 w484] -> w424
            frame False {
              # "Nincs hibaág"
              n92 = case shown="True" w442 {
                tunnel: [w458 w462] -> w450
                tunnel: w449 -> [w457 w463]
                tunnel: w448 -> [w456 w465]
                tunnel: w447 -> [_ w460]
                tunnel: w446 -> [w455 w464]
                tunnel: w445 -> [_ _]
                tunnel: w444 -> [w454 w466]
                tunnel: [w454 w466] -> w443
                tunnel: [FALSE w461] -> w441
                tunnel: w440 -> [_ _]
                tunnel: w439 -> [w451 w459]
                tunnel: [w451 w459] -> w438
                frame False {
                  # "Mérési hiba"
                  n93 = call-poly "Enqueue Message.vi"("error in (no error)"=w457, "Message Data"=w455, "Message"="Step Up PTR", "Message Queue"=w456) -> ("error out"=w458:errorcluster)  [unwired: 6 in, 1 out]
                }
                frame True {
                  # "Géphiba"
                  n94 = case shown="False" w460 {
                    selector: w460 -> [_ w478]
                    tunnel: [w477 w479] -> w462
                    tunnel: w463 -> [w476 w481]
                    tunnel: w465 -> [w475 w482]
                    tunnel: w464 -> [w469 w480]
                    tunnel: [TRUE w478] -> w461
                    frame False {
                      w468 = "ENGINE Jump" ("Command.Parancs")
                      w472 = T1 {"Thread ID"=0.0, "Mérésszám"="", "Mérés/Utasítás"="", "Command"={"Parancs"="", "Paraméter 1"="", "Paraméter 2"="", "Paraméter 3"="", "Paraméter 4"="", "Paraméter 5"="", "Eredmény"=""}, "Min"="", "Max"="", "Aktív?"=FALSE, "Log?"=FALSE, "Kiértékelés"=FALSE, "Etalon 1 exp"=FALSE, "Etalon 2 exp"=FALSE, "Etalon 3 exp"=FALSE, "Etalon 4 exp"=FALSE, "Etalon 5 exp"=FALSE}  # Teszt cluster
                      w471 = T3 {"Thread ID"=0, "Callback"="", "Data"=variant, "Error"={"status"=FALSE, "code"=0, "source"=""}}  # Message
                      n95 = Bundle By Name(cluster=w472, "Command.Parancs"=w468, "Command.Paraméter 1"="TESTER_ERROR") -> (w474:T1)
                      n96 = Bundle By Name(cluster=w471, "Thread ID"=w469, "Data"=w474) -> (w470:T3)
                      n97 = call-poly "Enqueue Message.vi"("error in (no error)"=w476, "Message Data"=w470, "Message"=w468, "Message Queue"=w475) -> ("error out"=w477:errorcluster)  [unwired: 6 in, 1 out]
                    }
                    frame True {
                      n98 = call-poly "Enqueue Message.vi"("error in (no error)"=w481, "Message Data"=w480, "Message"="Step Up PTR", "Message Queue"=w482) -> ("error out"=w479:errorcluster)  [unwired: 6 in, 1 out]
                    }
                  }
                }
              }
            }
            frame True {
              w484 = TRUE
              w491 = "ENGINE Jump" ("Command.Parancs")
              w494 = T1 {"Thread ID"=0.0, "Mérésszám"="", "Mérés/Utasítás"="", "Command"={"Parancs"="", "Paraméter 1"="", "Paraméter 2"="", "Paraméter 3"="", "Paraméter 4"="", "Paraméter 5"="", "Eredmény"=""}, "Min"="", "Max"="", "Aktív?"=FALSE, "Log?"=FALSE, "Kiértékelés"=FALSE, "Etalon 1 exp"=FALSE, "Etalon 2 exp"=FALSE, "Etalon 3 exp"=FALSE, "Etalon 4 exp"=FALSE, "Etalon 5 exp"=FALSE}  # Teszt cluster
              w493 = T3 {"Thread ID"=0, "Callback"="", "Data"=variant, "Error"={"status"=FALSE, "code"=0, "source"=""}}  # Message
              # "Van hibaág"
              n99 = Bundle By Name(cluster=w494, "Command.Parancs"=w491, "Command.Paraméter 1"=w486) -> (w495:T1)
              n100 = Bundle By Name(cluster=w493, "Thread ID"=w489, "Data"=w495) -> (w492:T3)
              n101 = call-poly "Enqueue Message.vi"("error in (no error)"=w488, "Message Data"=w492, "Message"=w491, "Message Queue"=w490) -> ("error out"=w487:errorcluster)  [unwired: 6 in, 1 out]
            }
          }
        }
        frame True {
          # "KÖVETKEZÕ TESZTRE UGRÁS"
          n102 = call-poly "Enqueue Message.vi"("error in (no error)"=w502, "Message Data"=w499, "Message"="Step Up PTR", "Message Queue"=w501) -> ("error out"=w503:errorcluster)  [unwired: 6 in, 1 out]
        }
      }
    }
    frame 4 {
      w513 = 4 ("length (rest)")
      n103 = Unbundle By Name(w508) -> ("Etalon 4 exp"=w507:bool)
      n104 = String Subset(string=w511, length (rest)=w513) -> (substring=w515:string)  [unwired: 1 in]
      n105 = Increment(x=w513) -> (x+1=w512:i32)
      n106 = Equal?(x=w507, y=w505) -> (x = y?=w506:bool)
      n107 = Equal?(x=w515, y="GOTO") -> (x = y?=w510:bool)
      n108 = String Subset(string=w511, offset (0)=w512) -> (substring=w509:string)  [unwired: 1 in]
      n109 = case shown="False" w506 {
        selector: w506 -> [w525 w596]
        tunnel: [w537 w603] -> w518
        tunnel: w522 -> [w536 w602]
        tunnel: w519 -> [w535 w601]
        tunnel: w520 -> [w533 w599]
        tunnel: w521 -> [w534 _]
        tunnel: [w531 w597] -> w523
        tunnel: w511 -> [w532 _]
        tunnel: w517 -> [w530 _]
        tunnel: [w529 FALSE] -> w516
        tunnel: w510 -> [w527 _]
        tunnel: w509 -> [w528 _]
        tunnel: w505 -> [w526 w597]
        tunnel: [w524 w596] -> w504
        frame False {
          # "KIÉRTÉKELÉS"
          n110 = case shown="True" w527 {
            tunnel: [w550 w587] -> w537
            tunnel: w536 -> [w549 w588]
            tunnel: w535 -> [w548 w590]
            tunnel: w534 -> [w547 _]
            tunnel: w533 -> [w546 w589]
            tunnel: w532 -> [w545 _]
            tunnel: w526 -> [w544 _]
            tunnel: [w543 w584] -> w531
            tunnel: w530 -> [w542 _]
            tunnel: [w541 FALSE] -> w529
            tunnel: w528 -> [w540 w586]
            tunnel: w525 -> [w539 _]
            tunnel: [w538 w584] -> w524
            frame False {
              # "Nincs hibaág"
              n111 = case shown="True" w542 {
                tunnel: [w558 w562] -> w550
                tunnel: w549 -> [w557 w563]
                tunnel: w548 -> [w556 w565]
                tunnel: w547 -> [_ w560]
                tunnel: w546 -> [w555 w564]
                tunnel: w545 -> [_ _]
                tunnel: w544 -> [w554 w566]
                tunnel: [w554 w566] -> w543
                tunnel: [FALSE w561] -> w541
                tunnel: w540 -> [_ _]
                tunnel: w539 -> [w551 w559]
                tunnel: [w551 w559] -> w538
                frame False {
                  # "Mérési hiba"
                  n112 = call-poly "Enqueue Message.vi"("error in (no error)"=w557, "Message Data"=w555, "Message"="Step Up PTR", "Message Queue"=w556) -> ("error out"=w558:errorcluster)  [unwired: 6 in, 1 out]
                }
                frame True {
                  # "Géphiba"
                  n113 = case shown="False" w560 {
                    selector: w560 -> [_ w578]
                    tunnel: [w577 w579] -> w562
                    tunnel: w563 -> [w576 w581]
                    tunnel: w565 -> [w575 w582]
                    tunnel: w564 -> [w569 w580]
                    tunnel: [TRUE w578] -> w561
                    frame False {
                      w568 = "ENGINE Jump" ("Command.Parancs")
                      w572 = T1 {"Thread ID"=0.0, "Mérésszám"="", "Mérés/Utasítás"="", "Command"={"Parancs"="", "Paraméter 1"="", "Paraméter 2"="", "Paraméter 3"="", "Paraméter 4"="", "Paraméter 5"="", "Eredmény"=""}, "Min"="", "Max"="", "Aktív?"=FALSE, "Log?"=FALSE, "Kiértékelés"=FALSE, "Etalon 1 exp"=FALSE, "Etalon 2 exp"=FALSE, "Etalon 3 exp"=FALSE, "Etalon 4 exp"=FALSE, "Etalon 5 exp"=FALSE}  # Teszt cluster
                      w571 = T3 {"Thread ID"=0, "Callback"="", "Data"=variant, "Error"={"status"=FALSE, "code"=0, "source"=""}}  # Message
                      n114 = Bundle By Name(cluster=w572, "Command.Parancs"=w568, "Command.Paraméter 1"="TESTER_ERROR") -> (w574:T1)
                      n115 = Bundle By Name(cluster=w571, "Thread ID"=w569, "Data"=w574) -> (w570:T3)
                      n116 = call-poly "Enqueue Message.vi"("error in (no error)"=w576, "Message Data"=w570, "Message"=w568, "Message Queue"=w575) -> ("error out"=w577:errorcluster)  [unwired: 6 in, 1 out]
                    }
                    frame True {
                      n117 = call-poly "Enqueue Message.vi"("error in (no error)"=w581, "Message Data"=w580, "Message"="Step Up PTR", "Message Queue"=w582) -> ("error out"=w579:errorcluster)  [unwired: 6 in, 1 out]
                    }
                  }
                }
              }
            }
            frame True {
              w584 = TRUE
              w591 = "ENGINE Jump" ("Command.Parancs")
              w594 = T1 {"Thread ID"=0.0, "Mérésszám"="", "Mérés/Utasítás"="", "Command"={"Parancs"="", "Paraméter 1"="", "Paraméter 2"="", "Paraméter 3"="", "Paraméter 4"="", "Paraméter 5"="", "Eredmény"=""}, "Min"="", "Max"="", "Aktív?"=FALSE, "Log?"=FALSE, "Kiértékelés"=FALSE, "Etalon 1 exp"=FALSE, "Etalon 2 exp"=FALSE, "Etalon 3 exp"=FALSE, "Etalon 4 exp"=FALSE, "Etalon 5 exp"=FALSE}  # Teszt cluster
              w593 = T3 {"Thread ID"=0, "Callback"="", "Data"=variant, "Error"={"status"=FALSE, "code"=0, "source"=""}}  # Message
              # "Van hibaág"
              n118 = Bundle By Name(cluster=w594, "Command.Parancs"=w591, "Command.Paraméter 1"=w586) -> (w595:T1)
              n119 = Bundle By Name(cluster=w593, "Thread ID"=w589, "Data"=w595) -> (w592:T3)
              n120 = call-poly "Enqueue Message.vi"("error in (no error)"=w588, "Message Data"=w592, "Message"=w591, "Message Queue"=w590) -> ("error out"=w587:errorcluster)  [unwired: 6 in, 1 out]
            }
          }
        }
        frame True {
          # "KÖVETKEZÕ TESZTRE UGRÁS"
          n121 = call-poly "Enqueue Message.vi"("error in (no error)"=w602, "Message Data"=w599, "Message"="Step Up PTR", "Message Queue"=w601) -> ("error out"=w603:errorcluster)  [unwired: 6 in, 1 out]
        }
      }
    }
    frame 5 {
      w613 = 4 ("length (rest)")
      n122 = Unbundle By Name(w608) -> ("Etalon 5 exp"=w607:bool)
      n123 = String Subset(string=w611, length (rest)=w613) -> (substring=w615:string)  [unwired: 1 in]
      n124 = Increment(x=w613) -> (x+1=w612:i32)
      n125 = Equal?(x=w607, y=w605) -> (x = y?=w606:bool)
      n126 = Equal?(x=w615, y="GOTO") -> (x = y?=w610:bool)
      n127 = String Subset(string=w611, offset (0)=w612) -> (substring=w609:string)  [unwired: 1 in]
      n128 = case shown="False" w606 {
        selector: w606 -> [w625 w696]
        tunnel: [w637 w703] -> w618
        tunnel: w622 -> [w636 w702]
        tunnel: w619 -> [w635 w701]
        tunnel: w620 -> [w633 w699]
        tunnel: w621 -> [w634 _]
        tunnel: [w631 w697] -> w623
        tunnel: w611 -> [w632 _]
        tunnel: w617 -> [w630 _]
        tunnel: [w629 FALSE] -> w616
        tunnel: w610 -> [w627 _]
        tunnel: w609 -> [w628 _]
        tunnel: w605 -> [w626 w697]
        tunnel: [w624 w696] -> w604
        frame False {
          # "KIÉRTÉKELÉS"
          n129 = case shown="True" w627 {
            tunnel: [w650 w687] -> w637
            tunnel: w636 -> [w649 w688]
            tunnel: w635 -> [w648 w690]
            tunnel: w634 -> [w647 _]
            tunnel: w633 -> [w646 w689]
            tunnel: w632 -> [w645 _]
            tunnel: w626 -> [w644 _]
            tunnel: [w643 w684] -> w631
            tunnel: w630 -> [w642 _]
            tunnel: [w641 FALSE] -> w629
            tunnel: w628 -> [w640 w686]
            tunnel: w625 -> [w639 _]
            tunnel: [w638 w684] -> w624
            frame False {
              # "Nincs hibaág"
              n130 = case shown="True" w642 {
                tunnel: [w658 w662] -> w650
                tunnel: w649 -> [w657 w663]
                tunnel: w648 -> [w656 w665]
                tunnel: w647 -> [_ w660]
                tunnel: w646 -> [w655 w664]
                tunnel: w645 -> [_ _]
                tunnel: w644 -> [w654 w666]
                tunnel: [w654 w666] -> w643
                tunnel: [FALSE w661] -> w641
                tunnel: w640 -> [_ _]
                tunnel: w639 -> [w651 w659]
                tunnel: [w651 w659] -> w638
                frame False {
                  # "Mérési hiba"
                  n131 = call-poly "Enqueue Message.vi"("error in (no error)"=w657, "Message Data"=w655, "Message"="Step Up PTR", "Message Queue"=w656) -> ("error out"=w658:errorcluster)  [unwired: 6 in, 1 out]
                }
                frame True {
                  # "Géphiba"
                  n132 = case shown="False" w660 {
                    selector: w660 -> [_ w678]
                    tunnel: [w677 w679] -> w662
                    tunnel: w663 -> [w676 w681]
                    tunnel: w665 -> [w675 w682]
                    tunnel: w664 -> [w669 w680]
                    tunnel: [TRUE w678] -> w661
                    frame False {
                      w668 = "ENGINE Jump" ("Command.Parancs")
                      w672 = T1 {"Thread ID"=0.0, "Mérésszám"="", "Mérés/Utasítás"="", "Command"={"Parancs"="", "Paraméter 1"="", "Paraméter 2"="", "Paraméter 3"="", "Paraméter 4"="", "Paraméter 5"="", "Eredmény"=""}, "Min"="", "Max"="", "Aktív?"=FALSE, "Log?"=FALSE, "Kiértékelés"=FALSE, "Etalon 1 exp"=FALSE, "Etalon 2 exp"=FALSE, "Etalon 3 exp"=FALSE, "Etalon 4 exp"=FALSE, "Etalon 5 exp"=FALSE}  # Teszt cluster
                      w671 = T3 {"Thread ID"=0, "Callback"="", "Data"=variant, "Error"={"status"=FALSE, "code"=0, "source"=""}}  # Message
                      n133 = Bundle By Name(cluster=w672, "Command.Parancs"=w668, "Command.Paraméter 1"="TESTER_ERROR") -> (w674:T1)
                      n134 = Bundle By Name(cluster=w671, "Thread ID"=w669, "Data"=w674) -> (w670:T3)
                      n135 = call-poly "Enqueue Message.vi"("error in (no error)"=w676, "Message Data"=w670, "Message"=w668, "Message Queue"=w675) -> ("error out"=w677:errorcluster)  [unwired: 6 in, 1 out]
                    }
                    frame True {
                      n136 = call-poly "Enqueue Message.vi"("error in (no error)"=w681, "Message Data"=w680, "Message"="Step Up PTR", "Message Queue"=w682) -> ("error out"=w679:errorcluster)  [unwired: 6 in, 1 out]
                    }
                  }
                }
              }
            }
            frame True {
              w684 = TRUE
              w691 = "ENGINE Jump" ("Command.Parancs")
              w694 = T1 {"Thread ID"=0.0, "Mérésszám"="", "Mérés/Utasítás"="", "Command"={"Parancs"="", "Paraméter 1"="", "Paraméter 2"="", "Paraméter 3"="", "Paraméter 4"="", "Paraméter 5"="", "Eredmény"=""}, "Min"="", "Max"="", "Aktív?"=FALSE, "Log?"=FALSE, "Kiértékelés"=FALSE, "Etalon 1 exp"=FALSE, "Etalon 2 exp"=FALSE, "Etalon 3 exp"=FALSE, "Etalon 4 exp"=FALSE, "Etalon 5 exp"=FALSE}  # Teszt cluster
              w693 = T3 {"Thread ID"=0, "Callback"="", "Data"=variant, "Error"={"status"=FALSE, "code"=0, "source"=""}}  # Message
              # "Van hibaág"
              n137 = Bundle By Name(cluster=w694, "Command.Parancs"=w691, "Command.Paraméter 1"=w686) -> (w695:T1)
              n138 = Bundle By Name(cluster=w693, "Thread ID"=w689, "Data"=w695) -> (w692:T3)
              n139 = call-poly "Enqueue Message.vi"("error in (no error)"=w688, "Message Data"=w692, "Message"=w691, "Message Queue"=w690) -> ("error out"=w687:errorcluster)  [unwired: 6 in, 1 out]
            }
          }
        }
        frame True {
          # "KÖVETKEZÕ TESZTRE UGRÁS"
          n140 = call-poly "Enqueue Message.vi"("error in (no error)"=w702, "Message Data"=w699, "Message"="Step Up PTR", "Message Queue"=w701) -> ("error out"=w703:errorcluster)  [unwired: 6 in, 1 out]
        }
      }
    }
  }
  "Kiértékelés" <- w15
  "error out" <- w9
  "Etalon Kiértékelés" <- w1
  "Abort" <- w2
